vi "LPT_List_Heuristic.vi"() -> ()   [LabVIEW 2013]
uses:
  Classes/OSSP_Problem.lvclass
  Classes/GanntChart_Class/Operation to Machine Job Tuple.vi
  Classes/GanntChart.lvclass
panel:
  out "Total Tardiness":u16
  in  "Problem Type":enum16{"Taillard", "Brucker", "Gueret Prins"}(ring)
  out "Makespan":u16
  out "Array 2":i32[](array[numeric])
  out "sorted array":cluster{"Numeric":u16, i32}[](array[cluster])
  out "Array":i32[](array[numeric])
  out "Processing Times":u16[][](array[numeric])
  out "output array":u16[](array[numeric])
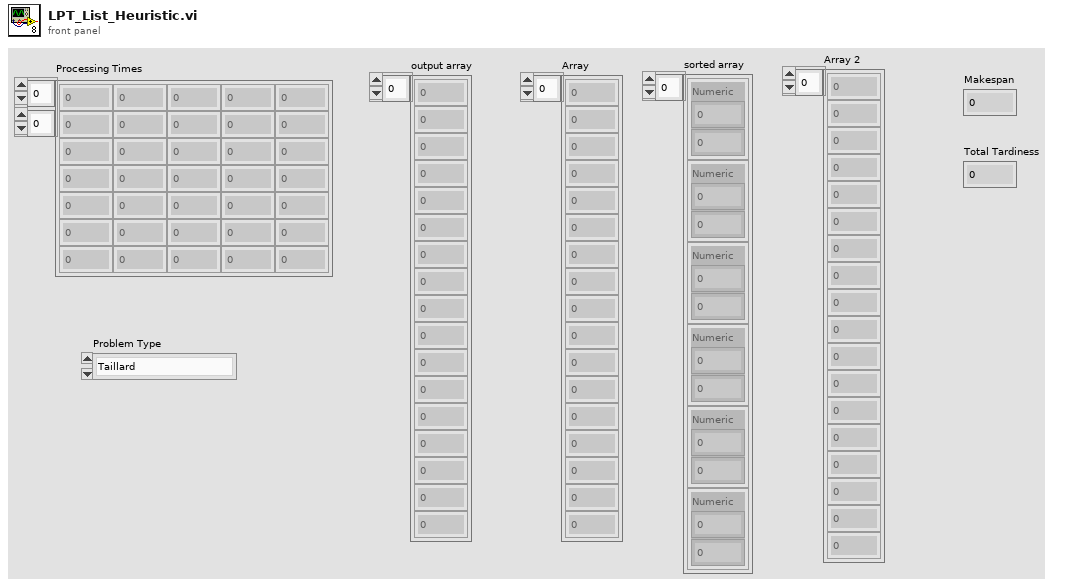
[diagram p1: front panel]
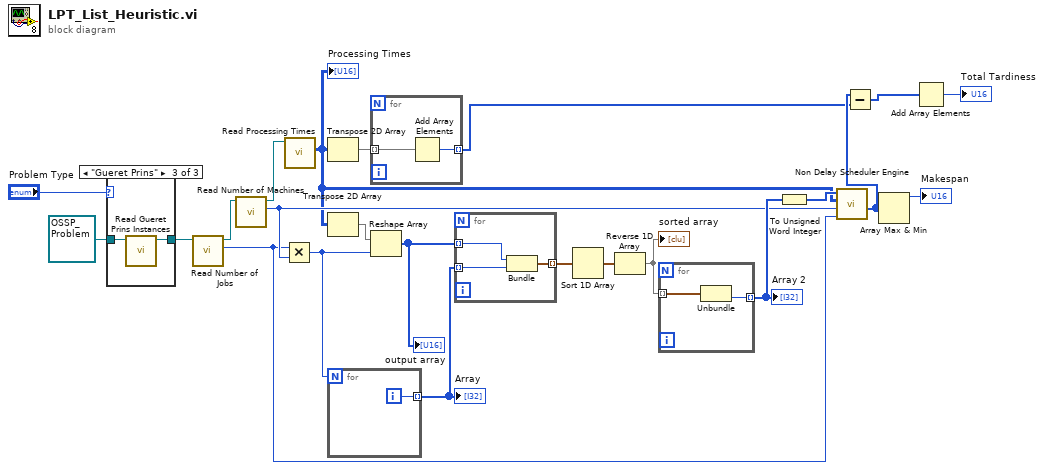
[diagram p0: block diagram]
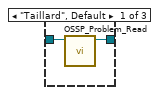
[diagram p2: hidden frame]
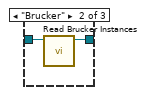
[diagram p3: hidden frame]
diagram:
  n1 = case shown="\"Gueret Prins\"" "Problem Type" {
    tunnel: refnum<class "OSSP_Problem.lvclass"> refnum ("OSSP_Problem.lvclass In") -> [w25 w27 w29]
    tunnel: [w24 w26 w28] -> w22
    frame "Taillard", Default {
      n2 = call "OSSP_Problem_Read.vi"("OSSP_Problem.lvclass In"=w25) -> ("OSSP_Problem.lvclass Out"=w24:refnum<class "OSSP_Problem.lvclass">)  [unwired: 7 in, 3 out]
    }
    frame "Brucker" {
      n3 = call "Read Brucker Instances.vi"("OSSP_Problem in"=w27) -> ("OSSP_Problem out"=w26:refnum<class "OSSP_Problem.lvclass">)  [unwired: 8 in, 2 out]
    }
    frame "Gueret Prins" {
      n4 = call "Read Gueret Prins Instances.vi"("OSSP_Problem in"=w29) -> ("OSSP_Problem out"=w28:refnum<class "OSSP_Problem.lvclass">)  [unwired: 8 in, 2 out]
    }
  }
  n5 = call-dynamic "Read Number of Jobs.vi"("OSSP_Problem in"=w22) -> ("Number of Jobs"=w9:i32, "OSSP_Problem out"=w21:refnum<class "OSSP_Problem.lvclass">)  [unwired: 8 in, 1 out]
  n6 = call-dynamic "Read Number of Machines.vi"("OSSP_Problem in"=w21) -> ("Number of Machines"=w10:i32, "OSSP_Problem out"=w20:refnum<class "OSSP_Problem.lvclass">)  [unwired: 8 in, 1 out]
  n7 = Multiply(x=w9, y=w10) -> (x*y=w18:i32)
  n8 = call-dynamic "Read Processing Times.vi"("OSSP_Problem in"=w20) -> ("Processing Times"=w5:u16[][])  [unwired: 8 in, 2 out]
  "Processing Times" <- w5
  n9 = Transpose 2D Array(2D array=w5) -> (transposed array=w6:u16[][])
  n10 = Transpose 2D Array(2D array=w5) -> (transposed array=w19:u16[][])
  n11 = for {
    N: w18 -> [_]
    tunnel: [w30] -> w16 mode=indexing
    i -> [w30]
  }
  "Array" <- w16
  n12 = for {
    tunnel: w6 -> [w32] mode=indexing
    tunnel: [w31] -> w3 mode=indexing
    n13 = Add Array Elements(numeric array=w32) -> (sum=w31:u16)
  }
  n14 = Reshape Array(w19, w18) -> (w17:u16[])
  "output array" <- w17
  n15 = for {
    tunnel: w17 -> [w35] mode=indexing
    tunnel: w16 -> [w34] mode=indexing
    tunnel: [w33] -> w15 mode=indexing
    n16 = Bundle("Numeric"=w35, w34) -> (w33:cluster{"Numeric":u16, i32})  [unwired: 1 in]
  }
  n17 = Sort 1D Array(array=w15) -> (sorted array=w14:cluster{"Numeric":u16, i32}[])
  n18 = Reverse 1D Array(array=w14) -> (reversed array=w13:cluster{"Numeric":u16, i32}[])
  "sorted array" <- w13
  n19 = for {
    tunnel: w13 -> [w37] mode=indexing
    tunnel: [w36] -> w12 mode=indexing
    n20 = Unbundle(w37) -> (w36:i32)  [unwired: 1 out]
  }
  "Array 2" <- w12
  n21 = To Unsigned Word Integer(number=w12) -> (unsigned 16bit integer=w11:u16[])
  n22 = call "Non Delay Scheduler Engine.vi"("Number of  Jobs"=w9, "Number of Machines"=w10, "Processing Times"=w5, "Schedule"=w11) -> ("Job Completion Times"=w4:u16[])  [unwired: 3 in, 4 out]
  n23 = Subtract(x=w4, y=w3) -> (x-y=w2:u16[])
  n24 = Array Max & Min(array=w4) -> (max value=→"Makespan":u16)  [unwired: 3 out]
  n25 = Add Array Elements(numeric array=w2) -> (sum=→"Total Tardiness":u16)
